vi "XML boolean.vi"(8 "tag":string, 11 "String":string) -> (3 "Boolean":bool)   [LabVIEW 2013]
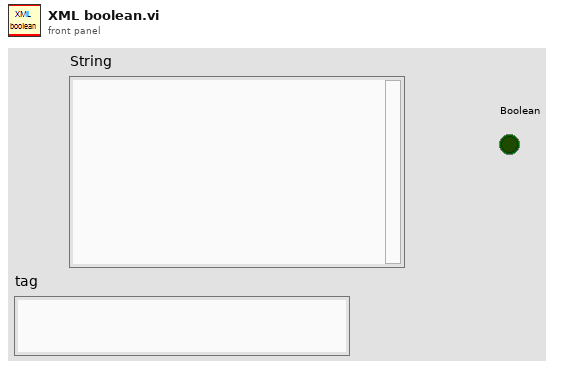
[diagram p1: front panel]
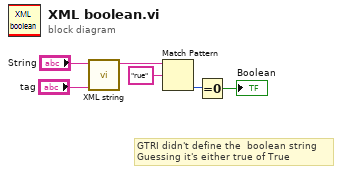
[diagram p0: block diagram]
diagram:
  # "GTRI didn't define the  boolean string\nGuessing it's either true of True"
  n1 = call "XML string.vi"("tag"="tag", "String"="String") -> ("string"=w4:string)  [unwired: 8 in, 1 out]
  n2 = Match Pattern(string=w4, regular expression="rue") -> (offset past match=w2:i32)  [unwired: 1 in, 3 out]
  n3 = Equal To 0?(x=w2) -> (x = 0?=→"Boolean":bool)
